vi "Set Field via Global Variables.vi"(1 "Rate (Oe/s)":dbl=10.0, 2 "Field":dbl) -> ()   [LabVIEW 2013]
uses:
  PPMS Global.vi
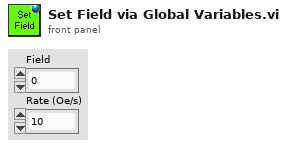
[diagram p1: front panel]
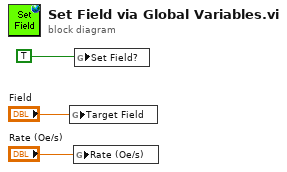
[diagram p0: block diagram]
diagram:
  n1 = global write "PPMS Global.vi" "Target Field"("Field") -> ()
  n2 = global write "PPMS Global.vi" "Rate (Oe/s)"("Rate (Oe/s)") -> ()
  n3 = global write "PPMS Global.vi" "Set Field?"(TRUE) -> ()
